vi "ProgG_010_MG.vi"() -> ()   [LabVIEW 2021]
panel:
  out "Objętość graniastosłupa [cm^3]":dbl=30.0
  in  "Wysokość graniastosłupa [cm]":dbl=5.0
  in  "c [cm]":dbl=5.0
  out "TAK - 1, NIE - 0":i32=1
  in  "b [cm]":dbl=4.0
  in  "a [cm]":dbl=3.0
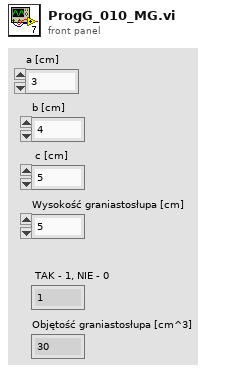
[diagram p1: front panel]
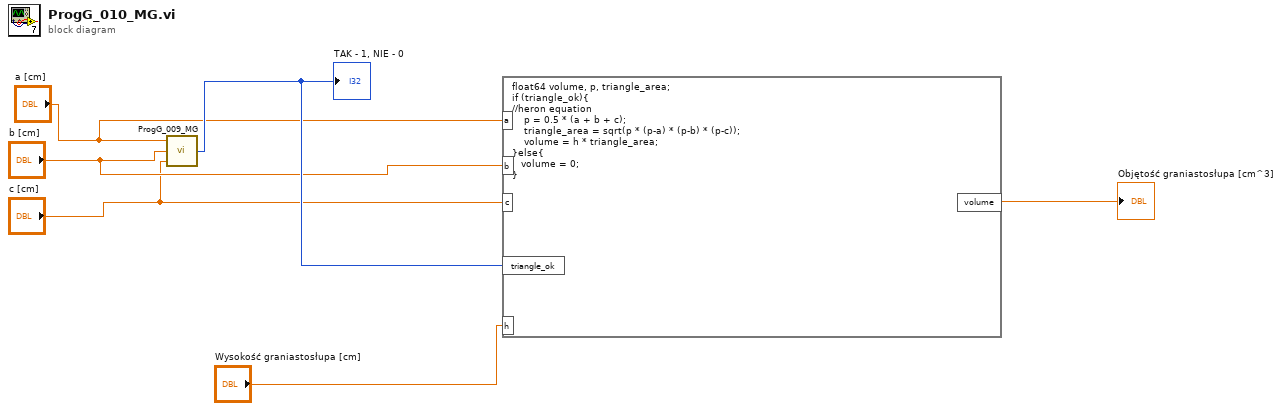
[diagram p0: block diagram]
diagram:
  n1 = call "ProgG_009_MG.vi"("c"="c [cm]", "b"="b [cm]", "a"="a [cm]") -> ("TAK - 1, NIE - 0"=w5:i32)
  "TAK - 1, NIE - 0" <- w5
  n2 = formula code="float64 volume, p, triangle_area;\nif (triangle_ok){\n//heron equation\n    p = 0.5 * (a + b + c);\n    triangle_area = sqrt(p * (p-a) * (p-b) * (p-c));\n    volume = h * triangle_area;\n}else{\n   volume = 0;\n}"("h"="Wysokość graniastosłupa [cm]", "triangle_ok"=w5, "a"="a [cm]", "b"="b [cm]", "c"="c [cm]") -> ("volume"=→"Objętość graniastosłupa [cm^3]":dbl)
